vi "Operation.vi"(8 "Error In":errorcluster, 11 "Subtract in":refnum<class "Subtract.lvclass">) -> (0 "Error Out":errorcluster, 2 "C":dbl, 3 "Subtract out":refnum<class "Subtract.lvclass">)   [LabVIEW 2023, in "Subtract.lvclass"]
doc: "The VI performs the subtraction operation for the two numbers and displays the output"
uses:
  Subtract.lvclass
  C:/Users/Ancy.Augustin/Downloads/LVOOPS DVR/LVOOPS DVR/Classes/Arithemtic Operation/Arithemetic Operation.lvclass
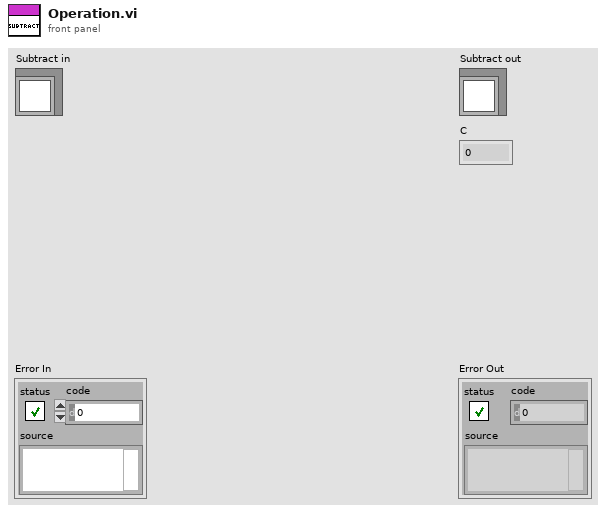
[diagram p1: front panel]
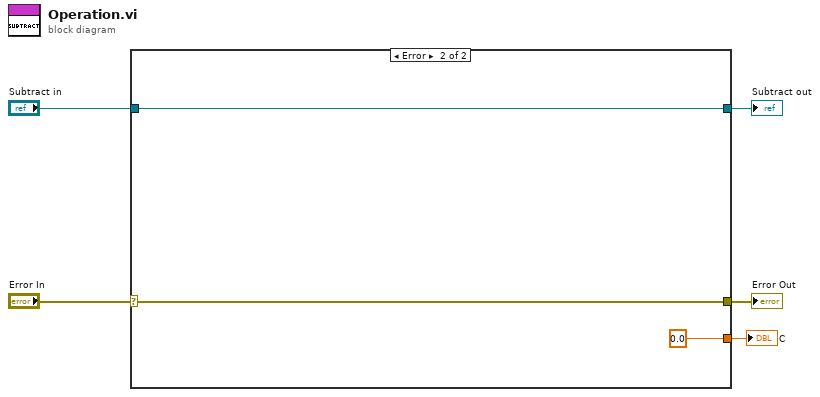
[diagram p0: block diagram]
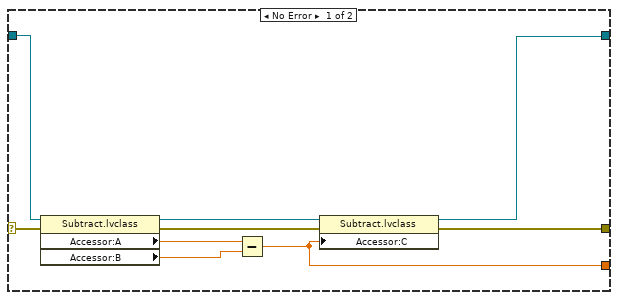
[diagram p2: hidden frame]
diagram:
  n1 = case shown="Error" "Error In" {
    selector: "Error In" -> [w14 w17]
    tunnel: [w9 w17] -> w4
    tunnel: [w6 w16] -> w2
    tunnel: "Subtract in" -> [w12 w16]
    tunnel: [w7 0.0] -> w1
    frame No Error {
      n2 = property class="Subtract.lvclass"(reference=w12, error in=w14) -> (reference out=w8:refnum<class "Subtract.lvclass">, error out=w13:errorcluster, "Accessor:A"=w11:dbl, "Accessor:B"=w10:dbl)
      n3 = Subtract(x=w11, y=w10) -> (x-y=w7:dbl)
      n4 = property class="Subtract.lvclass"(reference=w8, error in=w13, "Accessor:C"=w7) -> (reference out=w6:refnum<class "Subtract.lvclass">, error out=w9:errorcluster)
    }
    frame Error {
    }
  }
  "Error Out" <- w4
  "Subtract out" <- w2
  "C" <- w1
